vi "Render Tag.vi"(8 "Error In":errorcluster, 10 "Tag":refnum<class "Tag.lvclass">, 11 "Context In":refnum<class "Context.lvclass">) -> (0 "Error Out":errorcluster, 2 "Output":string, 3 "Context Out":refnum<class "Context.lvclass">)   [LabVIEW 2018, in "Toolkit.lvlib"]
uses:
  Toolkit.lvlib
  Nodes/Tag/Tag.lvclass
  Context/Context.lvclass
  Nodes/Tag/Tag.lvclass/Tag.ctl
  Data/String/String.lvclass
  Data/String/String.lvclass/String.ctl
  Data/Abstract/Abstract.lvclass
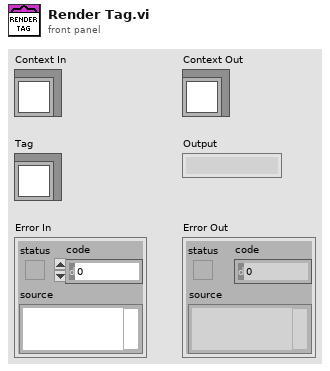
[diagram p1: front panel]
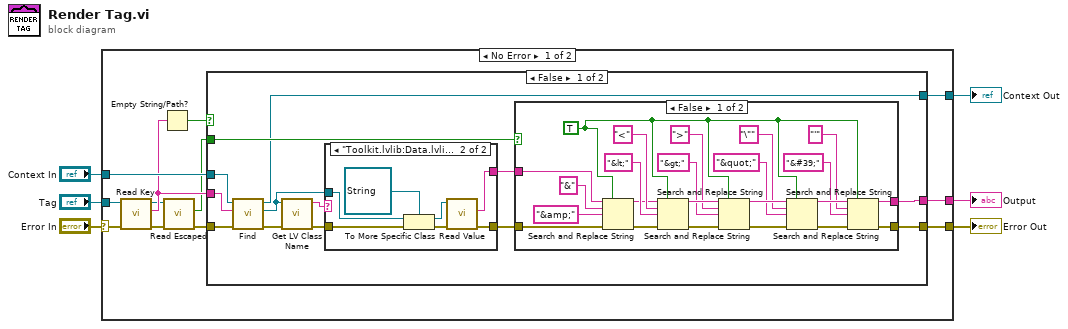
[diagram p0: block diagram]
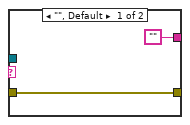
[diagram p2: hidden frame]
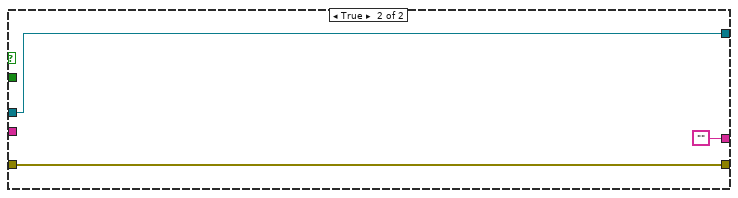
[diagram p4: hidden frame]
diagram:
  n1 = case shown="No Error" "Error In" {
    selector: "Error In" -> [w13 w70]
    tunnel: "Tag" -> [w12 _]
    tunnel: [w18 w70] -> w4
    tunnel: [w17 _] -> w3
    tunnel: "Context In" -> [w16 w69]
    tunnel: [w14 w69] -> w1
    frame No Error {
      n2 = call "Read Key.vi"("Error In"=w13, "Tag In"=w12) -> ("Error Out"=w9:errorcluster, "Key"=w11:string, "Tag Out"=w10:refnum<class "Tag.lvclass">)  [unwired: 7 in]
      n3 = Empty String/Path?(string/path=w11) -> (empty?=w15:bool)
      n4 = call "Read Escaped.vi"("Error In"=w9, "Tag In"=w10) -> ("Error Out"=w7:errorcluster, "Escaped"=w8:bool)  [unwired: 7 in, 1 out]
      n5 = case shown="False" w15 {
        tunnel: [w31 w68] -> w18
        tunnel: [w30 ""] -> w17
        tunnel: w8 -> [w29 _]
        tunnel: w16 -> [w24 w66]
        tunnel: w11 -> [w23 _]
        tunnel: w7 -> [w22 w68]
        tunnel: [w19 w66] -> w14
        frame False {
          n6 = call "Find.vi"("Error In"=w22, "Key"=w23, "Context In"=w24) -> ("Error Out"=w21:errorcluster, "Datum"=w20:refnum<class "Abstract.lvclass">, "Context Out"=w19:refnum<class "Context.lvclass">)  [unwired: 5 in, 1 out]
          n7 = call <vilib>:"Get LV Class Name.vi"("error in (no error)"=w21, "object"=w20) -> ("error out"=w27:errorcluster, "class name"=w28:string)  [unwired: 8 in]
          n8 = case shown="\"Toolkit.lvlib:Data.lvlib:String.lvclass\"" w28 {
            tunnel: w27 -> [w33 w40]
            tunnel: w20 -> [_ w38]
            tunnel: [w33 w35] -> w26
            tunnel: ["" w34] -> w25
            frame "", Default {
            }
            frame "Toolkit.lvlib:Data.lvlib:String.lvclass" {
              n9 = To More Specific Class(target class=refnum<class "String.lvclass"> refnum ("Toolkit.lvlib:Data.lvlib:String.lvclass"), reference=w38, error in=w40) -> (specific class reference=w36:refnum<class "String.lvclass">, error out=w37:errorcluster)
              n10 = call "Read Value.vi"("Error In"=w37, "String In"=w36) -> ("Error Out"=w35:errorcluster, "Value"=w34:string)  [unwired: 7 in, 1 out]
            }
          }
          n11 = case shown="False" w29 {
            tunnel: [w44 w64] -> w31
            tunnel: [w43 w65] -> w30
            tunnel: w26 -> [w42 w64]
            tunnel: w25 -> [w41 w65]
            frame False {
              w47 = TRUE ("replace all? (F)")
              n12 = Search and Replace String(replace all?=w47, input string=w41, search string="&", replace string="&amp;" ("replace string (\"\")"), error in=w42) -> (result string=w59:string, error out=w58:errorcluster)  [unwired: 3 in, 2 out]
              n13 = Search and Replace String(replace all?=w47, input string=w59, search string="<", replace string="&lt;" ("replace string (\"\")"), error in=w58) -> (result string=w56:string, error out=w57:errorcluster)  [unwired: 3 in, 2 out]
              n14 = Search and Replace String(replace all?=w47, input string=w56, search string=">", replace string="&gt;" ("replace string (\"\")"), error in=w57) -> (result string=w52:string, error out=w53:errorcluster)  [unwired: 3 in, 2 out]
              n15 = Search and Replace String(replace all?=w47, input string=w52, search string="\"" ("replace string (\"\")"), replace string="&quot;" ("replace string (\"\")"), error in=w53) -> (result string=w49:string, error out=w48:errorcluster)  [unwired: 3 in, 2 out]
              n16 = Search and Replace String(replace all?=w47, input string=w49, search string="'", replace string="&#39;" ("replace string (\"\")"), error in=w48) -> (result string=w43:string, error out=w44:errorcluster)  [unwired: 3 in, 2 out]
            }
            frame True {
            }
          }
        }
        frame True {
        }
      }
    }
    frame Error {
    }
  }
  "Error Out" <- w4
  "Output" <- w3
  "Context Out" <- w1
